vi "relay message to windows PC.vi"(8 "relay data":variant, 9 "relay message":string, 11 "RT Queues":T1) -> (3 "RT Queues out":T1)   [LabVIEW 2018]
uses:
  Type Defs/Queues cluster.ctl
  ICL-LabVIEW_General/Message Scheduler/message scheduler.lvclass
  ICL-LabVIEW_General/Incident logger/Incidents/Message/Message.lvclass
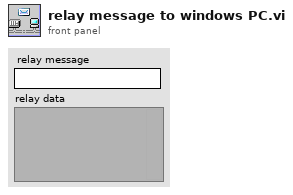
[diagram p1: front panel]
types:
  T1 = typedef "Queues cluster.ctl" = cluster{"RT Message":refnum<queue>, "RT Comms":refnum<queue>, "RT Data":refnum<queue>, "RT FIFO":refnum<queue>, "message scheduler":refnum<class "message scheduler.lvclass">}
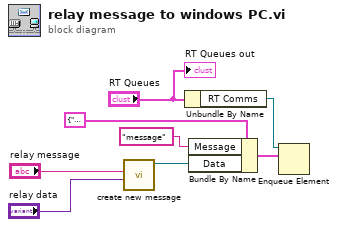
[diagram p0: block diagram]
diagram:
  n1 = call "create new message.vi"("Data"="relay data", "Message"="relay message") -> ("Message"=w1:refnum<class "Message.lvclass">)  [unwired: 8 in, 1 out]
  n2 = Unbundle By Name("RT Queues") -> ("RT Comms"=w7:refnum<queue>)
  n3 = Bundle By Name(cluster=cluster{"Message":string, "Data":variant} {"Message"="", "Data"=variant} ("element"), "Message"="message", "Data"=w1) -> (w5:cluster{"Message":string, "Data":variant})
  n4 = Enqueue Element(queue=w7, element=w5) -> ()  [unwired: 2 in, 3 out]
  "RT Queues out" <- "RT Queues"
